vi "Update Gauges.vi"(7 "Number of Sensors":i32=7) -> (10 "Analog Sensors":T1 {"Fuel Temp" scale=0.0..150.0 scale format="%#.1f"; "Flow(lbs/hr)" scale=0.0..1000.0 scale format="%#.1f"; "BP Monitor" scale=0.0..10.0 scale format="%#.1f"; "Bypass Pressure (psig)" scale=0.0..50.0 scale format="%#.1f"; "(Not Used)" scale=0.0..200.0 scale format="%#.1f"; "Back Pressure" scale=0.0..300.0 scale format="%#.1f"; "Diff. Pressure  (60 psid)" scale=0.0..60.0 scale format="%#.1f"; "Supply Pressure" scale=0.0..400.0 scale format="%#.1f"}, 13 "Actual Current":dbl)   [LabVIEW 2018]
uses:
  Controls/Gauge TDef.ctl
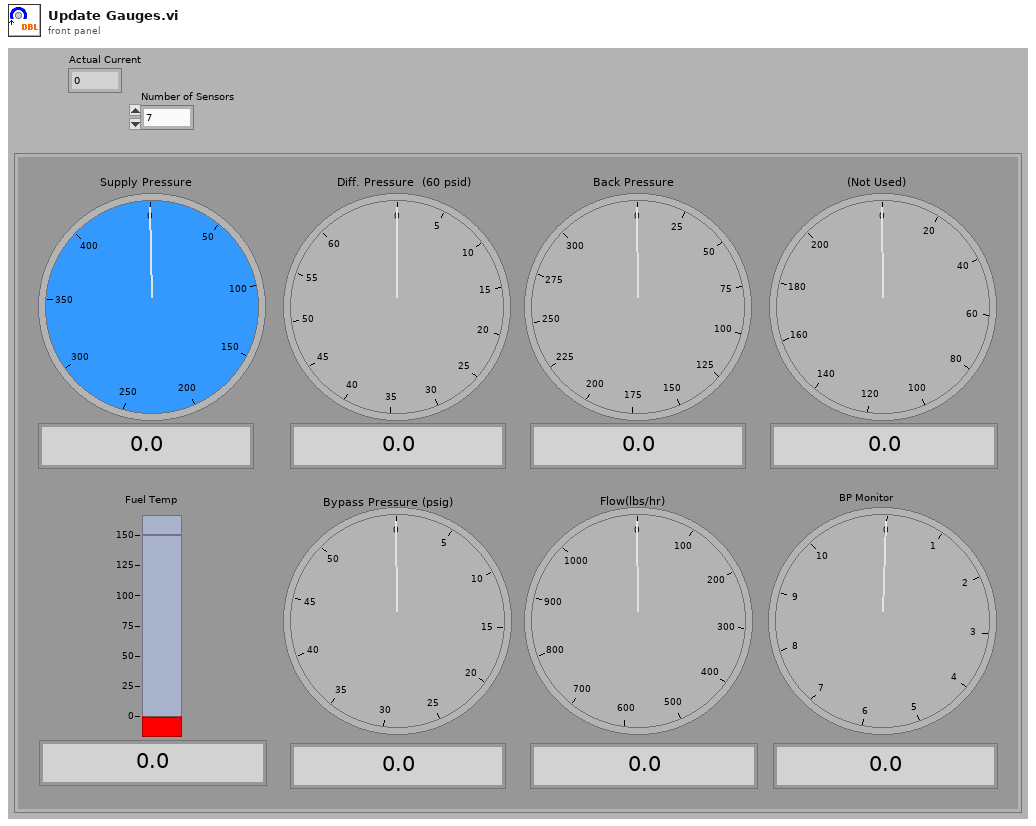
[diagram p1: front panel]
types:
  T1 = typedef "Gauge TDef.ctl" = cluster{"Flow(lbs/hr)":dbl, "Fuel Temp":dbl, "Supply Pressure":dbl, "Diff. Pressure  (60 psid)":dbl, "Back Pressure":dbl, "(Not Used)":dbl, "Bypass Pressure (psig)":dbl, "BP Monitor":dbl}
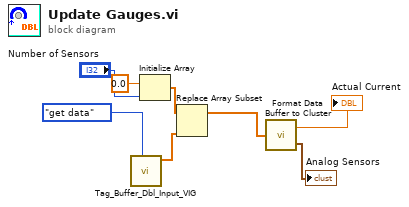
[diagram p0: block diagram]
diagram:
  n1 = call "Tag_Buffer_Dbl_Input_VIG.vi"("Operation"=enum16{"get data", "set data", "initialize"}."get data") -> ("tag_data_out"=w4:dbl[])  [unwired: 9 in, 1 out]
  n2 = Initialize Array(0.0, "Number of Sensors") -> (w5:dbl[])
  n3 = Replace Array Subset(array=w5, new element=w4) -> (w3:dbl[])  [unwired: 1 in]
  n4 = call "Format Data Buffer to Cluster.vi"("tag_data_out"=w3) -> ("Analog Sensors"=→"Analog Sensors":T1, "Actual Current"=→"Actual Current":dbl)
